vi "ZDS1104 Read.vi"(8 "错误输入":errorcluster, 9 "Function":u16(ring)=2 items=["Waveform Peak-Peak Value", "Waveform Amplitude Value", "Waveform Maximum", "Waveform Minimum", "Waveform Top Value", "Waveform Amplitude Base Value", "Rover Shoot", "Fover Shoot", "RPre Shoot", "FPre Shoot", "Waveform Amplitude Average(Display)", "Waveform Amplitude Average(Cycle)", "Waveform RMS(DC Display)", "Waveform RMS(DC Cycle)", "Waveform RMS(AC Display)", "Waveform RMS(AC Cycle)", "Waveform Adjust Mean", "Period", "Frequency", "Raising Time", "Fall Time", "Positive Pulse", "Negative Pulse", "Positive Duty", "Negative Duty", "Burst Width", "PulSetrain", "XMax", "XMin", "Setup Time", "Hold Time", "ShRatio", "Baud", "Raising Count", "Falling Count", "Positive Count", "Negtive Count", "Triger Count", "Area (Display)", "Area(Cycle)", "Positvie Area(Display)", "Positive Area(Cycle)", "Negtive Area(Display)", "Negtive Area(Cycle)"], 10 "Channel":u16(ring)=1 items=["Channel 1"=1, "Channel 2"=2, "Channel 3"=3, "Channel 4"=4], 11 "MyIndex":u8) -> (0 "error out":errorcluster caption="错误输出", 2 "ok?":bool, 3 "福值":dbl)   [LabVIEW 2015]
uses:
  ZhiYuan ZDS Series for TCP/ZhiYuan ZDS Series for TCP.lvlib
panel:
  out "VISA":refnum<visa-resource-name> caption="VISA资源名称输出"
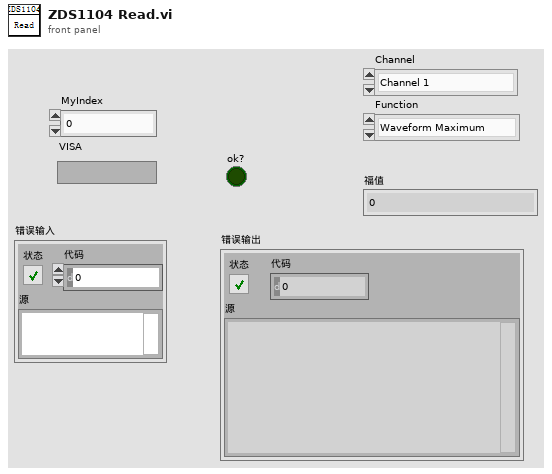
[diagram p1: front panel]
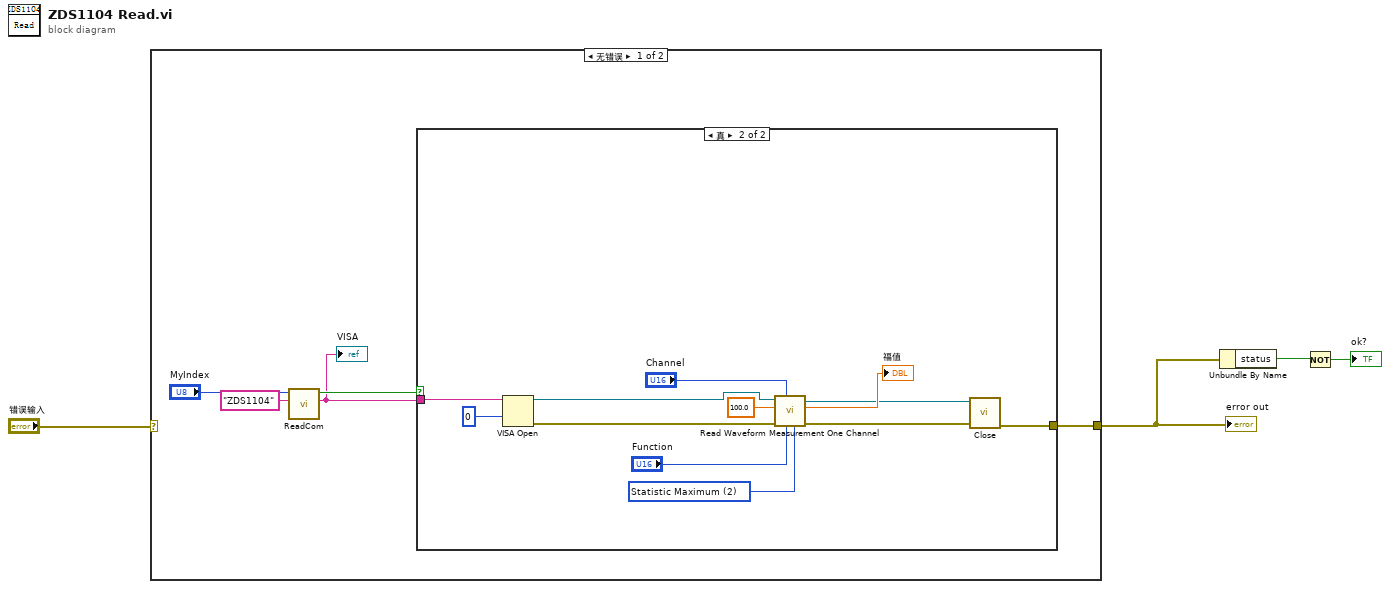
[diagram p0: block diagram]
diagram:
  n1 = case shown="无错误" "错误输入" {
    selector: "错误输入" -> [_ w22]
    tunnel: [w9 w22] -> w2
    frame No Error {
      n2 = call "ReadCom.vi"("仪器名称"="ZDS1104", "MyIndex"="MyIndex") -> ("COM"=w5:string, "OK?"=w6:bool)  [unwired: 7 in, 1 out]
      "VISA" <- w5
      n3 = case shown="真" w6 {
        tunnel: [_ w19] -> w9
        tunnel: w5 -> [_ w20]
        frame False {
        }
        frame True {
          w18 = u16 2 items=["Statistic Average", "Current Statistic Value", "Statistic Maximum", "Statistic Minimum", "Statistic Standard Deviation", "Counter"] ("Measurement Type (0: Statistic Average)")
          n4 = VISA Open(access mode=u32 0, VISA resource name=w20) -> (VISA resource name=w10:refnum<visa-resource-name>, error out=w13:errorcluster)  [unwired: 3 in]
          n5 = call "Read Waveform Measurement One Channel.vi"("Measurement Type (0: Statistic Average)"=w18, "Measurement Function (0: Falling Edge)"="Function", "Channel (1: Channel 1)"="Channel", "error in (no error)"=w13, "Timeout (1000 ms)"=100.0, "VISA resource name"=w10) -> ("error out"=w12:errorcluster, "Measurement"=→"福值":dbl, "VISA resource name out"=w11:refnum<visa-resource-name>)  [unwired: 3 in]
          n6 = call "Close.vi"("error in (no error)"=w12, "VISA resource name"=w11) -> ("error out"=w19:errorcluster)  [unwired: 9 in]
        }
      }
    }
    frame Error {
    }
  }
  "error out" <- w2
  n7 = Unbundle By Name(w2) -> ("status"=w4:bool)
  n8 = Not(x=w4) -> (.not. x?=→"ok?":bool)
